vi "Main.vi"() -> ()   [LabVIEW 2018]
uses:
  typedef/Parametros control.ctl
  <resource>/objmgr/daqmx.rc
  <vilib>/DAQmx/read.llb/DAQmx Read (Analog DBL 1Chan 1Samp).vi
  <vilib>/DAQmx/write.llb/DAQmx Write (Digital 1D Bool 1Chan 1Samp).vi
  <vilib>/DAQmx/write.llb/DAQmx Write (Counter Frequency 1Chan 1Samp).vi
  typedef/Selector control.ctl
panel:
  in  "Tiempo de ciclo":i32=20
  out "Image":T1(plugin-control)
  in  "Pause":bool
  in  "Acquire":bool
  in  "Ciclo de trabajo PWM":dbl=0.5000025
  in  "Device Name":tag="Dev6"
  in  "V. histeresis (grados)":dbl
  in  "Ganacias PID":T2
  out "Tiempo de ciclo (real)":u32
  out "Respuesta":cluster{"[0]":dbl, "[1]":dbl, "[2]":dbl}(graph)
  in  "Tipo de control":T3
  in  "Setpoint":dbl(knob) scale=-120.0..120.0
  out "PV":dbl(knob) caption="Variable de proceso" scale=-135.0..135.0
  in  "stop":bool
  in  "frequency":dbl=100.0 caption="Frecuencia PWM" format="%_6g"
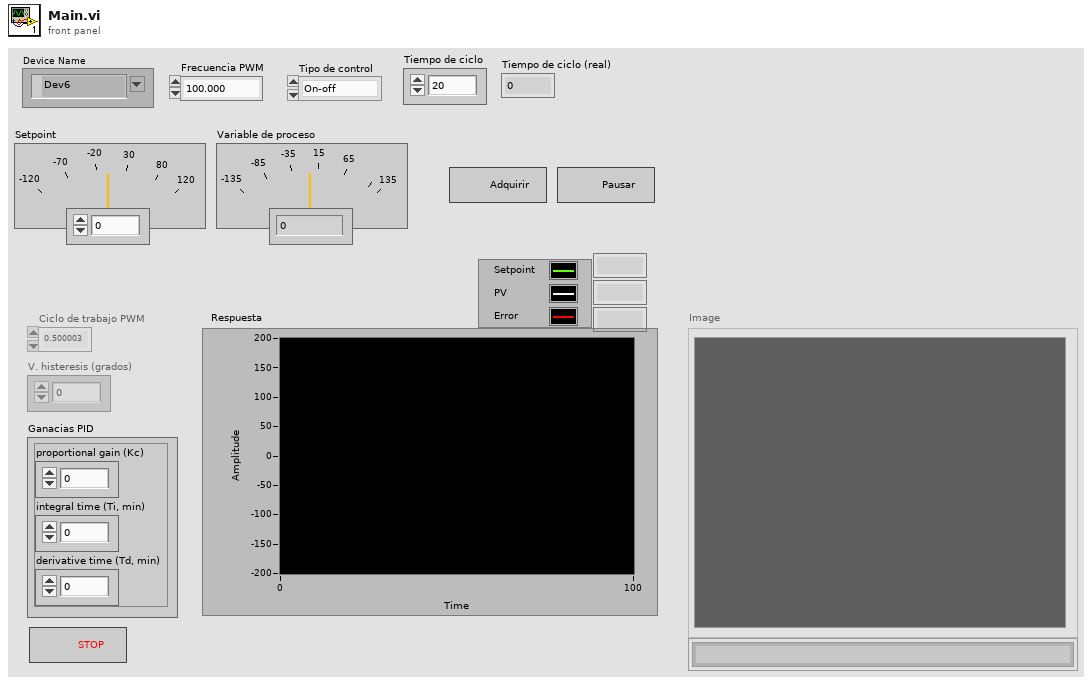
[diagram p1: front panel]
types:
  T1 = typedef "IMAQ Image.ctl" = refnum<image>
  T2 = cluster{"proportional gain (Kc)":dbl, "integral time (Ti, min)":dbl, "derivative time (Td, min)":dbl}
  T3 = typedef "Selector control.ctl" = enum16{"On-off", "On-off hist.", "PID"}
  T4 = typedef "Parametros control.ctl" = cluster{"Setpoint":dbl, "PV":dbl, "Frecuencia PWM":dbl, "Ciclo de trabajo PWM":dbl, "V. histeresis (grados)":dbl, "Ganacias PID":cluster{"proportional gain (Kc)":dbl, "integral time (Ti, min)":dbl, "derivative time (Td, min)":dbl}, "Ref array":refnum<vi>[]}
  T5 = typedef "Task list.ctl" = cluster{"PWM":refnum<k21>, "AI":refnum<k21>, "DO":refnum<k21>}
  T6 = enum8{"Enabled", "Disabled", "Disabled and Grayed Out"}[]
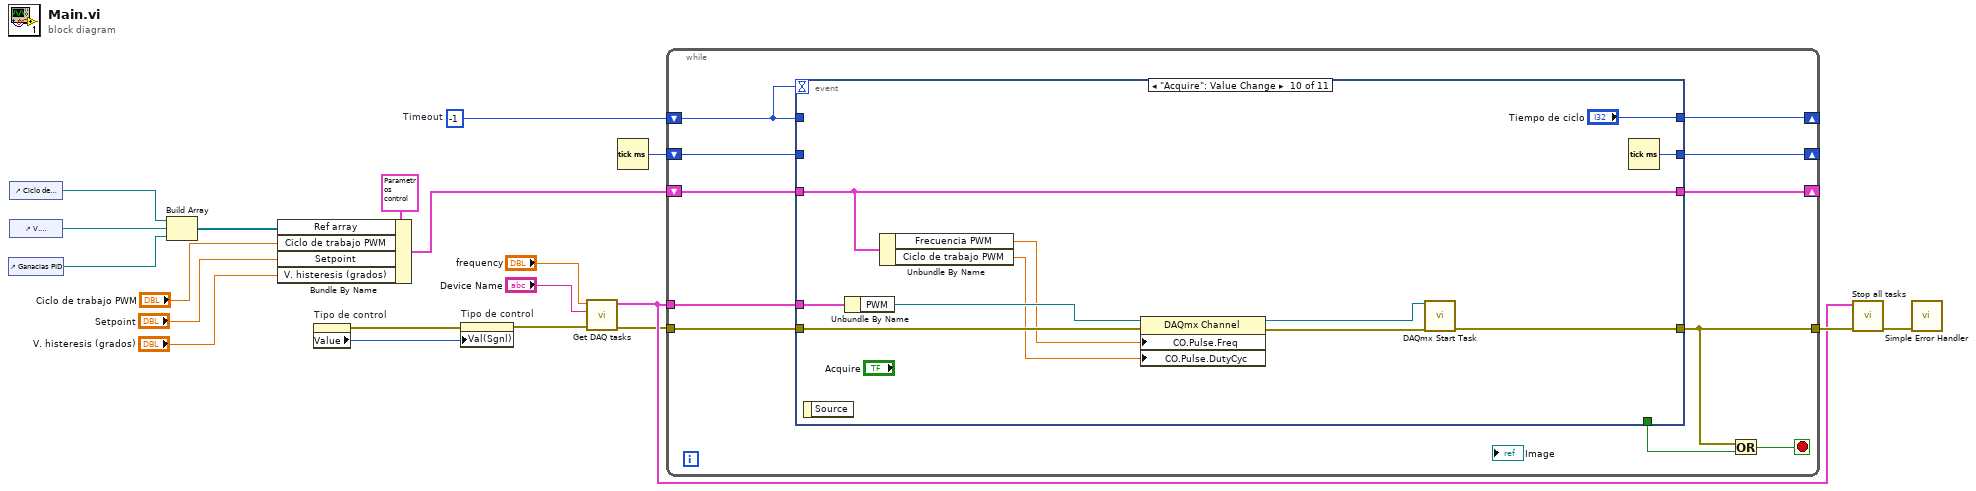
[diagram p0: block diagram]
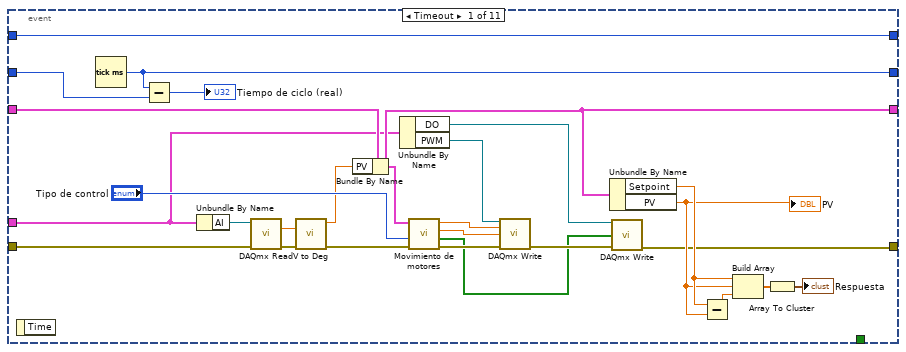
[diagram p2: hidden frame]
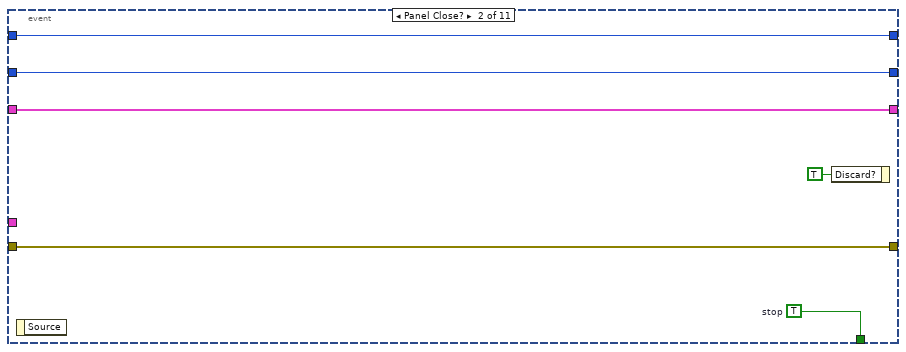
[diagram p3: hidden frame]
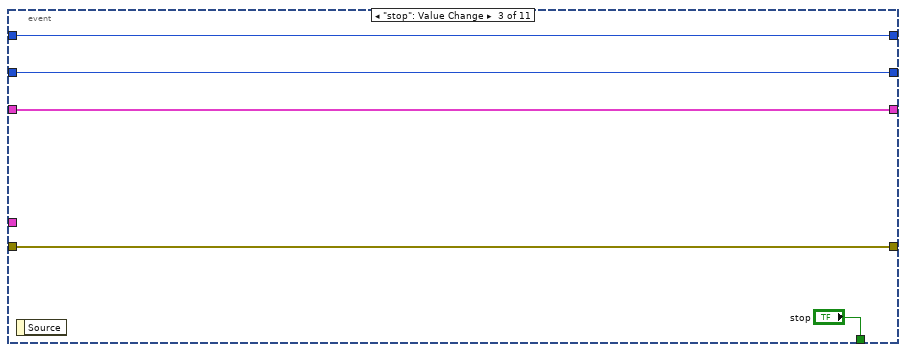
[diagram p4: hidden frame]
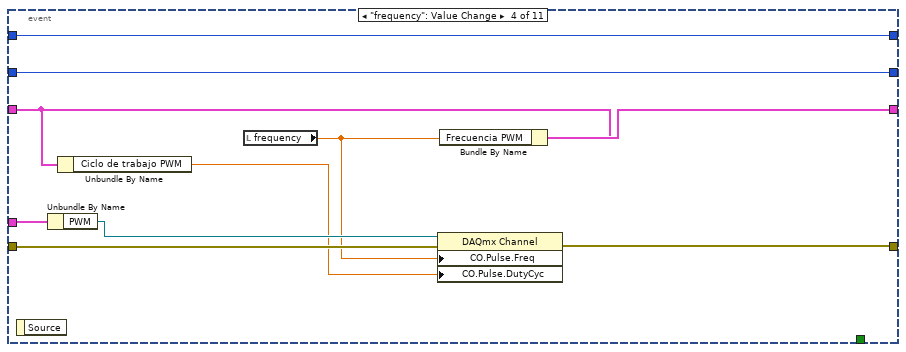
[diagram p5: hidden frame]
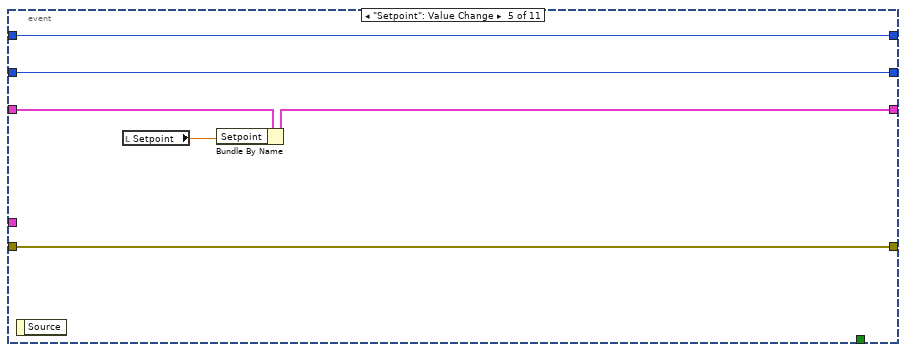
[diagram p6: hidden frame]
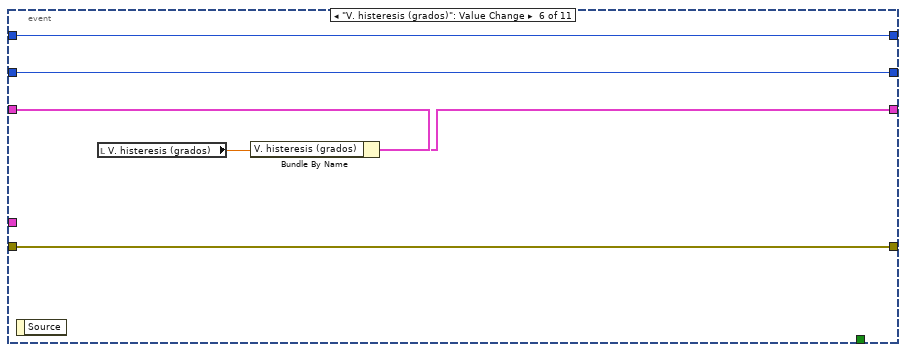
[diagram p7: hidden frame]
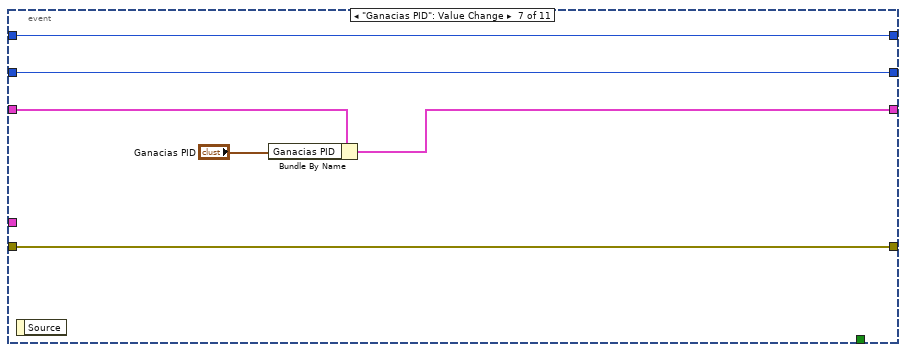
[diagram p8: hidden frame]
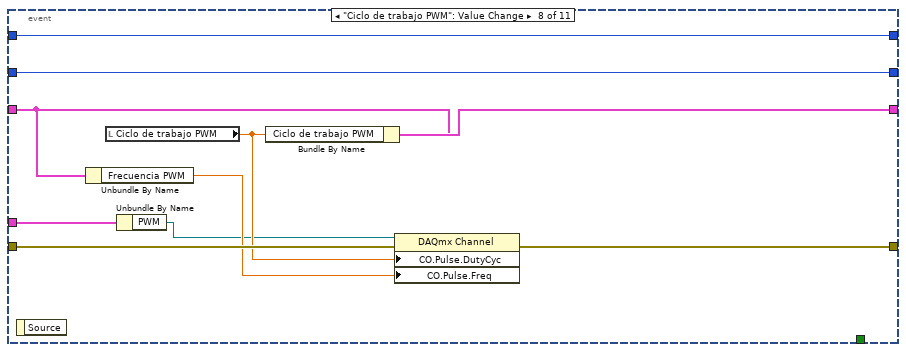
[diagram p9: hidden frame]
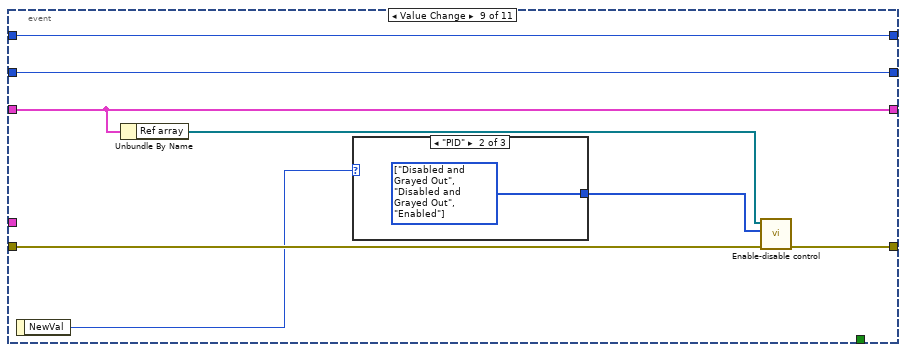
[diagram p10: hidden frame]
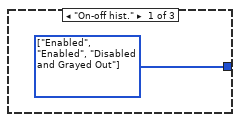
[diagram p11: hidden frame]
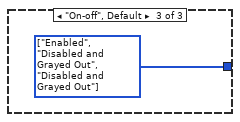
[diagram p12: hidden frame]
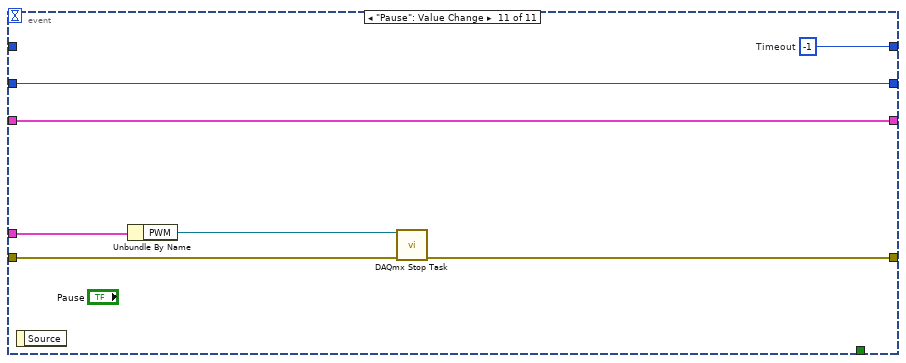
[diagram p13: hidden frame]
diagram:
  w15 = -1  # Timeout
  n1 = control-ref of="Ganacias PID"() -> (w12:refnum<vi>)
  n2 = control-ref of="Ciclo de trabajo PWM"() -> (w14:refnum<vi>)
  n3 = control-ref of="V. histeresis (grados)"() -> (w13:refnum<vi>)
  n4 = Build Array(w14, w13, w12) -> (w9:refnum<vi>[])
  n5 = Bundle By Name(cluster=T4 {"Setpoint"=0.0, "PV"=0.0, "Frecuencia PWM"=100.0, "Ciclo de trabajo PWM"=2.5e-06, "V. histeresis (grados)"=0.0, "Ganacias PID"={"proportional gain (Kc)"=1.0, "integral time (Ti, min)"=0.0, "derivative time (Td, min)"=0.0}, "Ref array"=[]} ("Parametros de control"), "Ref array"=w9, "Ciclo de trabajo PWM"="Ciclo de trabajo PWM", "Setpoint"="Setpoint", "V. histeresis (grados)"="V. histeresis (grados)") -> (w10:T4)
  n6 = property on="Tipo de control" class="Enum (strict)"() -> (error out=w5:errorcluster, "Value"=w6:T3)  [unwired: 2 in, 1 out]
  n7 = property on="Tipo de control" class="Enum (strict)"(error in=w5, "Val(Sgnl)"=w6) -> (error out=w7:errorcluster)  [unwired: 1 in, 1 out]
  n8 = call "Get DAQ tasks.vi"("error in"=w7, "Device Name"="Device Name", "frequency"="frequency") -> ("error out"=w8:errorcluster, "Task list"=w16:T5)  [unwired: 7 in]
  n9 = Tick Count (ms)() -> (millisecond timer value=w2:u32)
  n10 = while {
    tunnel: w8 -> [w30]
    tunnel: w16 -> [w31]
    tunnel: [w22] -> w18
    shift-right: [w28] -> _
    shift-left: w10 -> [w29]
    shift-right: [w26] -> _
    shift-left: w15 -> [w27]
    shift-right: [w24] -> _
    shift-left: w2 -> [w25]
    stop <- w21 stop-if-true
    n11 = event shown="[9] \"Acquire\": Value Change" {
      selector: _ -> [_ _ _ _ _ _ _ _ _ _ _]
      dyn-events: _ -> [_ _ _ _ _ _ _ _ _ _ _]
      timeout: w27 -> [_ _ _ _ _ _ _ _ _ _ _]
      tunnel: [_ w59 "stop" _ _ _ _ _ _ _ _] -> w23
      tunnel: w31 -> [w37 _ _ w77 _ _ _ w100 _ w129 w133]
      tunnel: w30 -> [w54 w64 w68 w75 w85 w91 w97 w105 w111 w126 w136]
      tunnel: [w34 w64 w68 w74 w85 w91 w97 w104 w110 w128 w134] -> w22
      tunnel: w29 -> [w50 w63 w66 w76 w84 w90 w96 w102 w113 w122 w135]
      tunnel: [w40 w63 w66 w79 w83 w89 w94 w106 w113 w122 w135] -> w28
      tunnel: w27 -> [w51 w62 w67 w78 w82 w88 w93 w107 w115 _ _]
      tunnel: [w51 w62 w67 w78 w82 w88 w93 w107 w115 "Tiempo de ciclo" w131] -> w26
      tunnel: w25 -> [w42 w61 w65 w70 w80 w87 w92 w98 w108 _ w130]
      tunnel: [w43 w61 w65 w70 w80 w87 w92 w98 w108 w119 w130] -> w24
      event Timeout {
        n12 = event-data() -> ()  [unwired: 1 in, 1 out]
        n13 = Tick Count (ms)() -> (millisecond timer value=w43:u32)
        n14 = Subtract(x=w43, y=w42) -> (x-y=→"Tiempo de ciclo (real)":u32)
        n15 = Unbundle By Name(w37) -> ("AI"=w52:refnum<k21>)
        n16 = call-poly <vilib>:"DAQmx Read.vi"("task/channels in"=w52, "error in"=w54) -> ("data"=w56:dbl, "error out"=w55:errorcluster)  [unwired: 11 in, 1 out]
        n17 = call "V to Deg.vi"("Voltaje de entrada (0-5V)"=w56, "error in (no error)"=w55) -> ("Angulo [-135, 135]"=w49:dbl, "error out"=w53:errorcluster)  [unwired: 7 in]
        n18 = Bundle By Name(cluster=w50, "PV"=w49) -> (w40:T4)
        n19 = Unbundle By Name(w37) -> ("DO"=w32:refnum<k21>, "PWM"=w36:refnum<k21>)
        n20 = call "Movimiento de motores.vi"("error in (no error)"=w53, "Tipo de control"="Tipo de control", "Parametros de control"=w40) -> ("error out"=w58:errorcluster, "DOs"=w33:bool[], "duty cycle"=w38:dbl, "frequency"=w39:dbl)  [unwired: 5 in]
        n21 = call-poly <vilib>:"DAQmx Write.vi"("task/channels in"=w36, "frequency"=w39, "duty cycle"=w38, "error in"=w58) -> ("error out"=w35:errorcluster)  [unwired: 9 in, 2 out]
        n22 = Unbundle By Name(w40) -> ("Setpoint"=w47:dbl, "PV"=w46:dbl)
        "PV" <- w46
        n23 = call-poly <vilib>:"DAQmx Write.vi"("task/channels in"=w32, "data"=w33, "error in"=w35) -> ("error out"=w34:errorcluster)  [unwired: 10 in, 2 out]
        n24 = Subtract(x=w47, y=w46) -> (x-y=w45:dbl)
        n25 = Build Array(w47, w46, w45) -> (w48:dbl[])
        n26 = Array To Cluster(array=w48) -> (cluster=→"Respuesta":cluster{"[0]":dbl, "[1]":dbl, "[2]":dbl})
      }
      event Panel Close? {
        w59 = TRUE  # stop
        n27 = event-data() -> ()  [unwired: 1 in, 1 out]
        n28 = event-data("Discard?"=TRUE) -> ()  [unwired: 1 in, 1 out]
      }
      event "stop": Value Change {
        n29 = event-data() -> ()  [unwired: 1 in, 1 out]
      }
      event "frequency": Value Change {
        n30 = event-data() -> ()  [unwired: 1 in, 1 out]
        n31 = Unbundle By Name(w77) -> ("PWM"=w73:refnum<k21>)
        n32 = Unbundle By Name(w76) -> ("Ciclo de trabajo PWM"=w71:dbl)
        n33 = local read "frequency"() -> (w72:dbl)
        n34 = property class="DAQmx Channel"(reference=w73, error in=w75, "CO.Pulse.Freq"=w72, "CO.Pulse.DutyCyc"=w71) -> (error out=w74:errorcluster)  [unwired: 1 out]
        n35 = Bundle By Name(cluster=w76, "Frecuencia PWM"=w72) -> (w79:T4)
      }
      event "Setpoint": Value Change {
        n36 = event-data() -> ()  [unwired: 1 in, 1 out]
        n37 = local read "Setpoint"() -> (w81:dbl)
        n38 = Bundle By Name(cluster=w84, "Setpoint"=w81) -> (w83:T4)
      }
      event "V. histeresis (grados)": Value Change {
        n39 = event-data() -> ()  [unwired: 1 in, 1 out]
        n40 = local read "V. histeresis (grados)"() -> (w86:dbl)
        n41 = Bundle By Name(cluster=w90, "V. histeresis (grados)"=w86) -> (w89:T4)
      }
      event "Ganacias PID": Value Change {
        n42 = event-data() -> ()  [unwired: 1 in, 1 out]
        n43 = Bundle By Name(cluster=w96, "Ganacias PID"="Ganacias PID") -> (w94:T4)
      }
      event "Ciclo de trabajo PWM": Value Change {
        n44 = event-data() -> ()  [unwired: 1 in, 1 out]
        n45 = Unbundle By Name(w102) -> ("Frecuencia PWM"=w101:dbl)
        n46 = local read "Ciclo de trabajo PWM"() -> (w103:dbl)
        n47 = Unbundle By Name(w100) -> ("PWM"=w99:refnum<k21>)
        n48 = Bundle By Name(cluster=w102, "Ciclo de trabajo PWM"=w103) -> (w106:T4)
        n49 = property class="DAQmx Channel"(reference=w99, error in=w105, "CO.Pulse.DutyCyc"=w103, "CO.Pulse.Freq"=w101) -> (error out=w104:errorcluster)  [unwired: 1 out]
      }
      event Value Change {
        n50 = event-data() -> ("NewVal"=w109:T3)  [unwired: 1 in]
        n51 = Unbundle By Name(w113) -> ("Ref array"=w112:refnum<vi>[])
        n52 = case shown="\"PID\"" w109 {
          tunnel: [w116 w117 w118] -> w114
          frame "On-off hist." {
            w116 = T6 [enum."Enabled", enum."Enabled", enum."Disabled and Grayed Out"] items=["Enabled", "Disabled", "Disabled and Grayed Out"] ("Status")
          }
          frame "PID" {
            w117 = T6 [enum."Disabled and Grayed Out", enum."Disabled and Grayed Out", enum."Enabled"] items=["Enabled", "Disabled", "Disabled and Grayed Out"] ("Status")
          }
          frame "On-off", Default {
            w118 = T6 [enum."Enabled", enum."Disabled and Grayed Out", enum."Disabled and Grayed Out"] items=["Enabled", "Disabled", "Disabled and Grayed Out"] ("Status")
          }
        }
        n53 = call "Enable-disable control.vi"("error in"=w111, "Status"=w114, "Ref array"=w112) -> ("error out"=w110:errorcluster)  [unwired: 8 in]
      }
      event "Acquire": Value Change {
        n54 = event-data() -> ()  [unwired: 1 in, 1 out]
        n55 = Unbundle By Name(w129) -> ("PWM"=w124:refnum<k21>)
        n56 = Unbundle By Name(w122) -> ("Frecuencia PWM"=w121:dbl, "Ciclo de trabajo PWM"=w120:dbl)
        n57 = property class="DAQmx Channel"(reference=w124, error in=w126, "CO.Pulse.Freq"=w121, "CO.Pulse.DutyCyc"=w120) -> (reference out=w123:refnum<k21>, error out=w125:errorcluster)
        n58 = call <vilib>:"DAQmx Start Task.vi"("task/channels in"=w123, "error in"=w125) -> ("error out"=w128:errorcluster)  [unwired: 12 in, 1 out]
        n59 = Tick Count (ms)() -> (millisecond timer value=w119:u32)
      }
      event "Pause": Value Change {
        w131 = -1  # Timeout
        n60 = event-data() -> ()  [unwired: 1 in, 1 out]
        n61 = Unbundle By Name(w133) -> ("PWM"=w132:refnum<k21>)
        n62 = call <vilib>:"DAQmx Stop Task.vi"("task/channels in"=w132, "error in"=w136) -> ("error out"=w134:errorcluster)  [unwired: 12 in, 1 out]
      }
    }
    n63 = Or(x=w22, y=w23) -> (x .or. y?=w21:bool)
  }
  n64 = call "Stop all tasks.vi"("error in"=w18, "Task list"=w16) -> ("error out"=w17:errorcluster)  [unwired: 9 in]
  n65 = call <vilib>:"Simple Error Handler.vi"("error in (no error)"=w17) -> ()  [unwired: 4 in, 5 out]
